vi "Poly Set Map Add New Type.vi"(6 "Selector Name":string, 7 "Poly Ref Map":T3, 8 "error in (no error)":errorcluster, 9 "Menu Name":string, 10 "New Library Path":path, 11 "Poly Map Set in":T1) -> (0 "error out":errorcluster, 3 "Poly Map Set out":T1)   [LabVIEW 2020]
uses:
  _td_map_PolyInstanceInfo.ctl
  _td_cluster_InstanceInfo.ctl
  _td_map_PolyRef.ctl
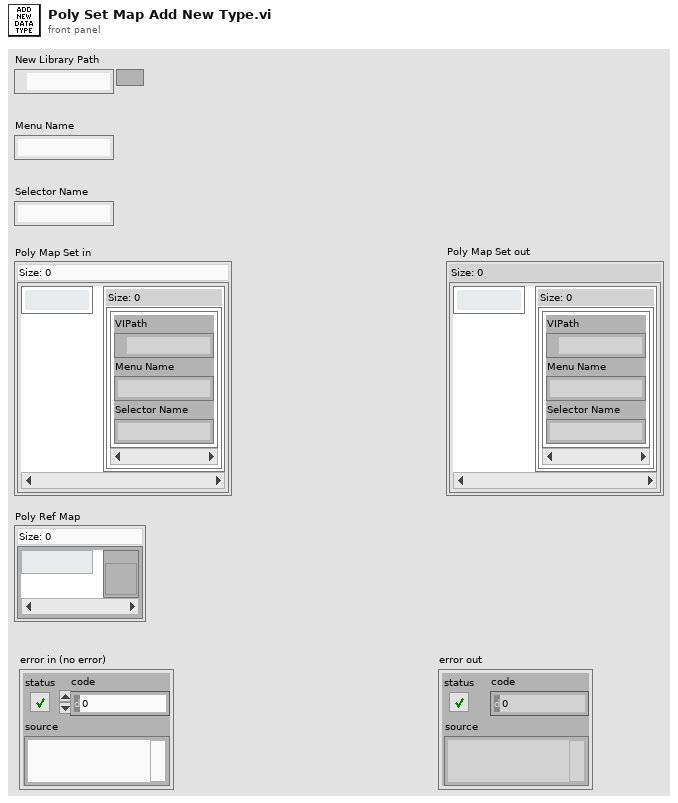
[diagram p1: front panel]
types:
  T1 = typedef "_td_map_PolyInstanceInfo.ctl" = map{string, set{T2}}
  T2 = typedef "_td_cluster_InstanceInfo.ctl" = cluster{"VIPath":path, "Menu Name":string, "Selector Name":string}
  T3 = typedef "_td_map_PolyRef.ctl" = map{string, refnum<vi>}
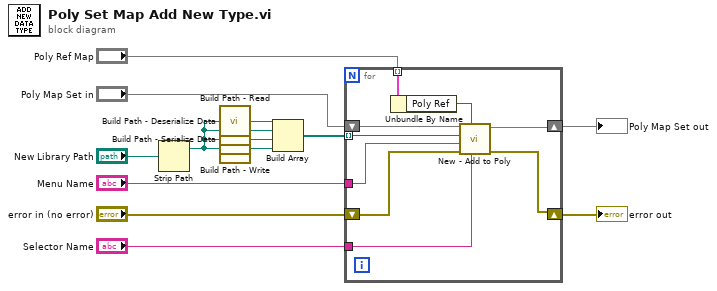
[diagram p0: block diagram]
diagram:
  n1 = Strip Path(path="New Library Path") -> (stripped path=w10:path)  [unwired: 1 out]
  n2 = call "Build Path - Deserialize Data.vi"("Directory"=w10) -> ("Path to Deserialize Data.vi"=w14:path)
  n3 = call "Build Path - Read.vi"("Directory"=w10) -> ("Path to Read.vi"=w13:path)
  n4 = call "Build Path - Serialize Data.vi"("Directory"=w10) -> ("Path to Serialize Data.vi"=w12:path)
  n5 = call "Build Path - Write.vi"("Directory"=w10) -> ("Path to Write.vi"=w11:path)
  n6 = Build Array(w14, w13, w12, w11) -> (w8:path[])
  n7 = for {
    tunnel: w8 -> [w19] mode=indexing
    tunnel: "Poly Ref Map" -> [w23] mode=indexing
    shift-right: [w20] -> w2
    shift-left: "Poly Map Set in" -> [w21]
    tunnel: "Menu Name" -> [w18]
    tunnel: "Selector Name" -> [w16]
    shift-right: [w15] -> w1
    shift-left: "error in (no error)" -> [w17]
    n8 = Unbundle By Name(w23) -> ("Poly Ref"=w22:refnum<vi>)
    n9 = call "New - Add to Poly.vi"("Selector Name"=w16, "Poly Ref"=w22, "error in (no error)"=w17, "Menu Name"=w18, "Path to VI"=w19, "Poly Map Set in"=w21) -> ("error out"=w15:errorcluster, "Poly Map Set out"=w20:T1)  [unwired: 4 in]
  }
  "Poly Map Set out" <- w2
  "error out" <- w1
